vi "Calculate Pad Scale.vi"(10 "Pad width":sgl, 11 "Length Y":sgl) -> (0 "Z Offset":sgl, 1 "Scale Z":sgl, 2 "Y Translation":sgl, 3 "Scale Y":sgl)   [LabVIEW 2017, in "NI_Robotics_Simulator.lvlib" / "ODESimulator_LinearConveyor.lvclass"]
uses:
  <vilib>/robotics/Simulator/Robot Factory/Conveyor/Linear/ODESimulator_LinearConveyor.lvclass
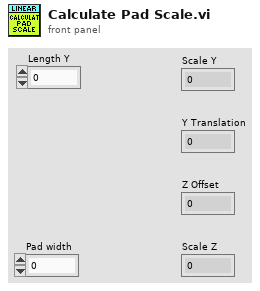
[diagram p1: front panel]
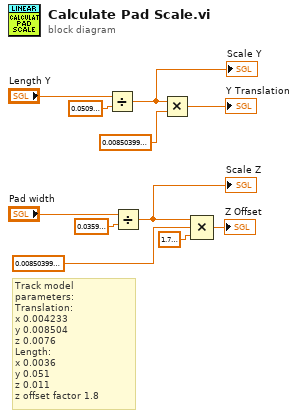
[diagram p0: block diagram]
diagram:
  # "Track model parameters:\nTranslation:\nx 0.004233\ny 0.008504\nz 0.0076\nLength:\nx 0.0036\ny 0.051\nz 0.011\nz offset factor 1.8"
  n1 = Divide(x="Length Y", y=sgl 0.051 ("x")) -> (x/y=w8:sgl)
  "Scale Y" <- w8
  n2 = Divide(x="Pad width", y=sgl 0.036 ("x")) -> (x/y=w5:sgl)
  "Scale Z" <- w5
  n3 = Multiply(x=w8, y=sgl 0.008504 ("Y")) -> (x*y=→"Y Translation":sgl)
  n4 = Compound Arithmetic op=MULTIPLY(w5, sgl 0.008504 ("Y"), sgl 1.8 ("value")) -> (→"Z Offset":sgl)
